vi "get remaining time budget.vi"(8 "error in":errorcluster, 10 "dt":u32=1, 11 "timing source in":refnum<class "usec timing source.lvclass">) -> (0 "error out":errorcluster, 2 "budget (ns)":u64, 3 "timing source out":refnum<class "usec timing source.lvclass">)   [LabVIEW 2013, in "usec timing source.lvclass"]
uses:
  usec timing source.lvclass
  usec timing source.lvclass/usec timing source.ctl
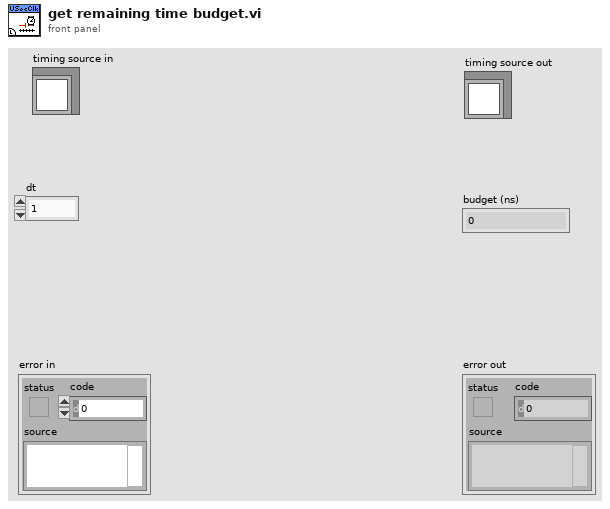
[diagram p1: front panel]
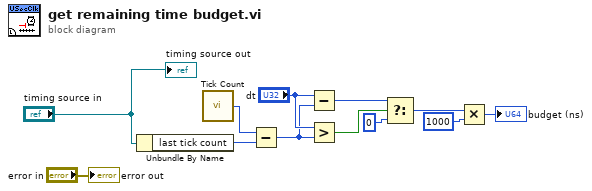
[diagram p0: block diagram]
diagram:
  n1 = Unbundle By Name("timing source in") -> ("last tick count"=w11:u32)
  n2 = call "Tick Count"() -> ("Tick Count(uSec)"=w10:u32)
  n3 = Subtract(x=w10, y=w11) -> (x-y=w7:u32)
  n4 = Subtract(x="dt", y=w7) -> (x-y=w6:u32)
  n5 = Greater?(x="dt", y=w7) -> (0:w9:bool)
  n6 = Select(t=w6, s=w9, f=u32 0) -> (s? t:f=w4:u32)
  n7 = Multiply(x=w4, y=u32 1000) -> (x*y=→"budget (ns)":u32)
  "error out" <- "error in"
  "timing source out" <- "timing source in"
